vi "SetDefaultHeaders_Core.vi"(8 "error in (no error)":errorcluster, 10 "Default Headers ([JSON])":T1[](array[typedef]), 11 "LabVIEWHTTPClient_NET in":refnum<class "HttpClient_NET.lvclass">) -> (0 "error out":errorcluster, 3 "LabVIEWHTTPClient_NET out":refnum<class "HttpClient_NET.lvclass">)   [LabVIEW 2018, in "REST Client_NET.lvlib" / "REST Client_NET.lvclass"]
doc: "<b> </b> <b> </b>\nHttpClient_NET\nJustin Young - Viviota\nCopyright (c) 2021\nLicense: BSD"
uses:
  REST Client_NET.lvclass
  <vilib>/addons/_JKI.lib/REST Client/classes/REST Client/HTTP Header.ctl
  LabVIEWHTTPClient_NET/HttpClient_NET.lvclass
  HttpHeaders_Request/HttpHeaders_Request.lvclass
  <vilib>/addons/_JKI.lib/REST Client/classes/REST Client/REST Client.lvclass
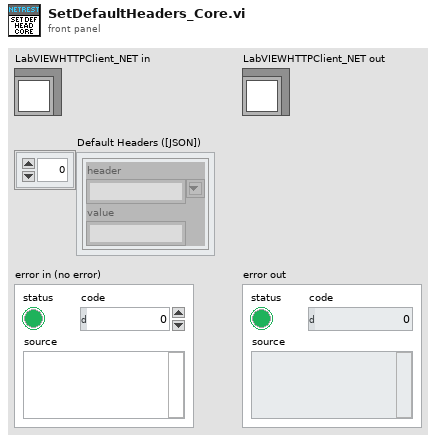
[diagram p1: front panel]
types:
  T1 = typedef "REST Client.lvlib/REST Client.lvclass/HTTP Header.ctl" = cluster{"header":string, "value":string}
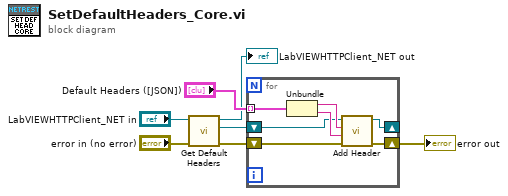
[diagram p0: block diagram]
diagram:
  n1 = call "Get Default Headers.vi"("error in (no error)"="error in (no error)", "LabVIEWHTTPClient_NET in"="LabVIEWHTTPClient_NET in") -> ("error out"=w7:errorcluster, "DefaultRequest Headers"=w6:refnum<class "HttpHeaders_Request.lvclass">, "LabVIEWHTTPClient_NET out"=→"LabVIEWHTTPClient_NET out":refnum<class "HttpClient_NET.lvclass">)  [unwired: 7 in]
  n2 = for {
    tunnel: "Default Headers ([JSON])" -> [w14] mode=indexing
    shift-right: [w10] -> _
    shift-left: w6 -> [w11]
    shift-right: [w8] -> w1
    shift-left: w7 -> [w9]
    n3 = Unbundle(w14) -> ("header"=w12:string, "value"=w13:string)
    n4 = call-dynamic "Add Header.vi"("error in (no error)"=w9, "Value"=w13, "Name"=w12, "HTTPHeaders_NET in"=w11) -> ("error out"=w8:errorcluster, "HTTPHeaders_NET out"=w10:refnum<class "HttpHeaders_Request.lvclass">)  [unwired: 6 in]
  }
  "error out" <- w1
